vi "New Targets Update from Targets Message.vi"(2 "error in":errorcluster, 3 "Targets Message":T2, 4 "Current Time (ms)":dbl) -> (0 "error out":errorcluster, 1 "Targets Update":T1)   [LabVIEW 2016]
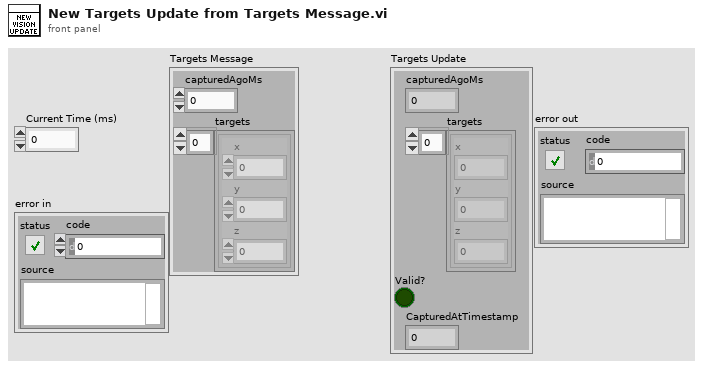
[diagram p1: front panel]
types:
  T1 = cluster{"capturedAgoMs":i32, "targets":cluster{"x":dbl, "y":dbl, "z":dbl}[], "Valid?":bool, "CapturedAtTimestamp":dbl}
  T2 = cluster{"capturedAgoMs":i32, "targets":cluster{"x":dbl, "y":dbl, "z":dbl}[]}
  T3 = cluster{"capturedAgoMs":i32, "targets":cluster{"X":dbl, "Y":dbl, "Z":dbl}[], "Valid?":bool, "CapturedAtTimestamp":dbl}
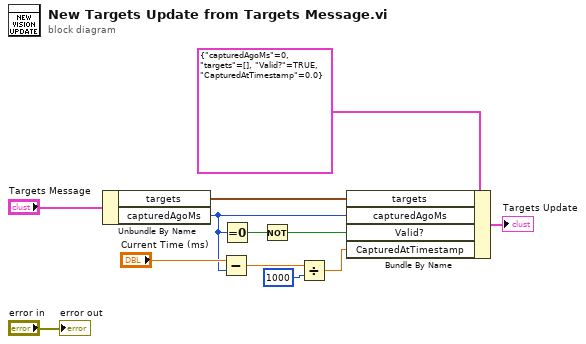
[diagram p0: block diagram]
diagram:
  n1 = Unbundle By Name("Targets Message") -> ("targets"=w5:cluster{"x":dbl, "y":dbl, "z":dbl}[], "capturedAgoMs"=w3:i32)
  n2 = Subtract(x="Current Time (ms)", y=w3) -> (x-y=w9:dbl)
  n3 = Equal To 0?(x=w3) -> (x = 0?=w11:bool)
  n4 = Not(x=w11) -> (.not. x?=w4:bool)
  n5 = Divide(x=w9, y=1000) -> (x/y=w2:dbl)
  n6 = Bundle By Name(cluster=T3 {"capturedAgoMs"=0, "targets"=[], "Valid?"=TRUE, "CapturedAtTimestamp"=0.0}, "targets"=w5, "capturedAgoMs"=w3, "Valid?"=w4, "CapturedAtTimestamp"=w2) -> (→"Targets Update":T3)
  "error out" <- "error in"
